vi "Send_command1.vi"(10 "string in":string, 11 "VISA Refnum in":refnum<visa-resource-name>) -> (3 "string out":string)   [LabVIEW 2013]
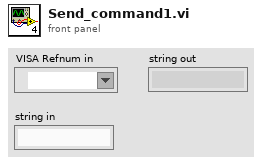
[diagram p1: front panel]
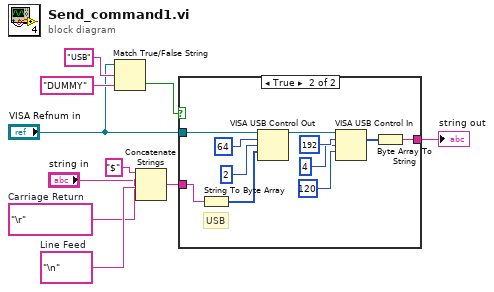
[diagram p0: block diagram]
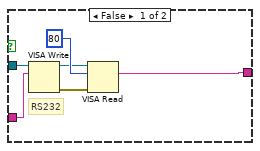
[diagram p2: hidden frame]
diagram:
  w7 = "\n"  # Line Feed
  w6 = "\r"  # Carriage Return
  n1 = Match True/False String(2:"DUMMY", 3:"USB", 4:"VISA Refnum in") -> (0:w9:bool)  [unwired: 1 out]
  n2 = Concatenate Strings("$", "string in", w6, w7) -> (w3:string)
  n3 = case shown="True" w9 {
    tunnel: [w14 w18] -> w2
    tunnel: w3 -> [w13 w27]
    tunnel: "VISA Refnum in" -> [w11 w17]
    frame False {
      # "RS232"
      n4 = VISA Write(VISA resource name=w11, write buffer=w13) -> (VISA resource name out=w15:refnum<visa-resource-name>, error out=w12:errorcluster)  [unwired: 1 in, 1 out]
      n5 = VISA Read(VISA resource name=w15, byte count=u32 80, error in (no error)=w12) -> (read buffer=w14:string)  [unwired: 3 out]
    }
    frame True {
      # "USB"
      n6 = String To Byte Array(string=w27) -> (unsigned byte array=w24:u8[])
      n7 = VISA USB Control Out(0:w17, 5:i16 64 ("request type"), 7:i16 2 ("request"), 9:w24) -> (4:w23:refnum<visa-resource-name>)  [unwired: 1 in, 3 out]
      n8 = VISA USB Control In(0:w23, 5:i16 192 ("request type"), 7:i16 4 ("request"), 9:u16 120 ("length (0)")) -> (6:w19:u8[])  [unwired: 1 in, 4 out]
      n9 = Byte Array To String(unsigned byte array=w19) -> (string=w18:string)
    }
  }
  "string out" <- w2
